vi "TEST_PP_Auto_Read.vi"() -> ()   [LabVIEW 2023]
uses:
  <vilib>/Rock Robotics/WPI/ThirdParty/MJansen/PathPlanner/TypeDef/PathPlannerTrajectoryState.ctl
  <vilib>/Rock Robotics/WPI/ThirdParty/JAS_Junk/TrajLib/TypeDef/TRANSLATION2D.ctl
  <vilib>/Rock Robotics/WPI/ThirdParty/JAS_Junk/TrajLib/TypeDef/ROTATION2D.ctl
  <vilib>/Rock Robotics/WPI/ThirdParty/MJansen/PathPlanner/TypeDef/PathPlannerPathConstraints.ctl
  <vilib>/Rock Robotics/WPI/ThirdParty/MJansen/PathPlanner/TypeDef/PathPlannerCommandUtil.ctl
  <vilib>/Rock Robotics/WPI/ThirdParty/MJansen/PathPlanner/ENum/PathPlanner_CommandUtilType_ENUM.ctl
  <vilib>/Rock Robotics/WPI/ThirdParty/MJansen/PathPlanner/TypeDef/PathPlannerEventMarker.ctl
  <vilib>/Rock Robotics/WPI/ThirdParty/JAS_Junk/TrajLib/VI/Util_GetTime_U32.vi
  <vilib>/Rock Robotics/WPI/ThirdParty/JAS_Junk/TrajLib/VI/BoolCmd_Recv_Internal.vi
  <vilib>/Utility/error.llb/Clear Errors.vi
  <vilib>/Rock Robotics/WPI/ThirdParty/JAS_Junk/TrajLib/Pose2d_New_TRRO.vi
  <vilib>/Rock Robotics/WPI/ThirdParty/MJansen/PathPlanner/VI/PathPlanner_EventMarker_ShouldTrigger.vi
  <vilib>/Rock Robotics/WPI/ThirdParty/JAS_Junk/TrajLib/VI/BoolCmd_ObtainQueue.vi
  <vilib>/Rock Robotics/WPI/ThirdParty/JAS_Junk/TrajLib/Translation2d_GetDistance.vi
  <vilib>/Rock Robotics/WPI/ThirdParty/JAS_Junk/TrajLib/Pose2d_getTranslation.vi
  <vilib>/Rock Robotics/WPI/ThirdParty/JAS_Junk/TrajLib/Util_CalcDist.vi
  <vilib>/Rock Robotics/WPI/ThirdParty/JAS_Junk/TrajLib/VI/Util_GetTime_U64.vi
  <vilib>/Rock Robotics/Network Tables/NT Write Number.vi
  <vilib>/Rock Robotics/Network Tables/NT Read Number.vi
  <vilib>/Rock Robotics/WPI/ThirdParty/MJansen/PathPlanner/PathPlanner24.lvlib
  <vilib>/Rock Robotics/WPI/ThirdParty/JAS_Junk/TrajLib/Trajectory_Library.lvlib
panel:
  out "time":dbl
  out "FPGA_Time_Seconds":dbl
  out "pathName":string
  out "size(s)":i32
  out "#Shoot":dbl
  out "EventMarkers":T1[](array[typedef]) {"lastRobotPos"."Y" format="%14.3f"; "lastRobotPos"."X" format="%14.3f"; "markerPos"."Y" format="%14.3f"; "markerPos"."X" format="%14.3f"}
  out "Req_Shoot_2":bool
  out "Req_Shoot_1":bool
  out "Auto Command":T3
  out "PathPlannerState":T5={"TimeSeconds"=0.0, "VelocityMPS"=0.0, "AccerationMpsSq"=0.0, "HeadingAngularVelRadPerSec"=0.0, "PositionMeters"={"X"=0.0, "Y"=1.0}, "Heading"={"VALUE"=0.0, "COS"=1.0, "SIN"=0.0}, "TargetHolonomicRotation"={"VALUE"=0.0, "COS"=1.0, "SIN"=0.0}, "CurvatureRadPerMeter"=0.0, "PathPlannerConstraints"={"MaxVelocityMps;"=0.0, "MaxAccelerationMpsSq;"=0.0, "MaxAngularVelRadPsEc;"=0.0, "MaxAngularAccRadPSecSq"=0.0, "Exists"=FALSE}, "DeltaPos"=0.0} {"TargetHolonomicRotation"."SIN" format="%13.4f"; "TargetHolonomicRotation"."COS" format="%13.4f"; "TargetHolonomicRotation"."VALUE" format="%13.4f"; "Heading"."SIN" format="%13.4f"; "Heading"."COS" format="%13.4f"; "Heading"."VALUE" format="%13.4f"; "PositionMeters"."Y" format="%14.3f"; "PositionMeters"."X" format="%14.3f"}
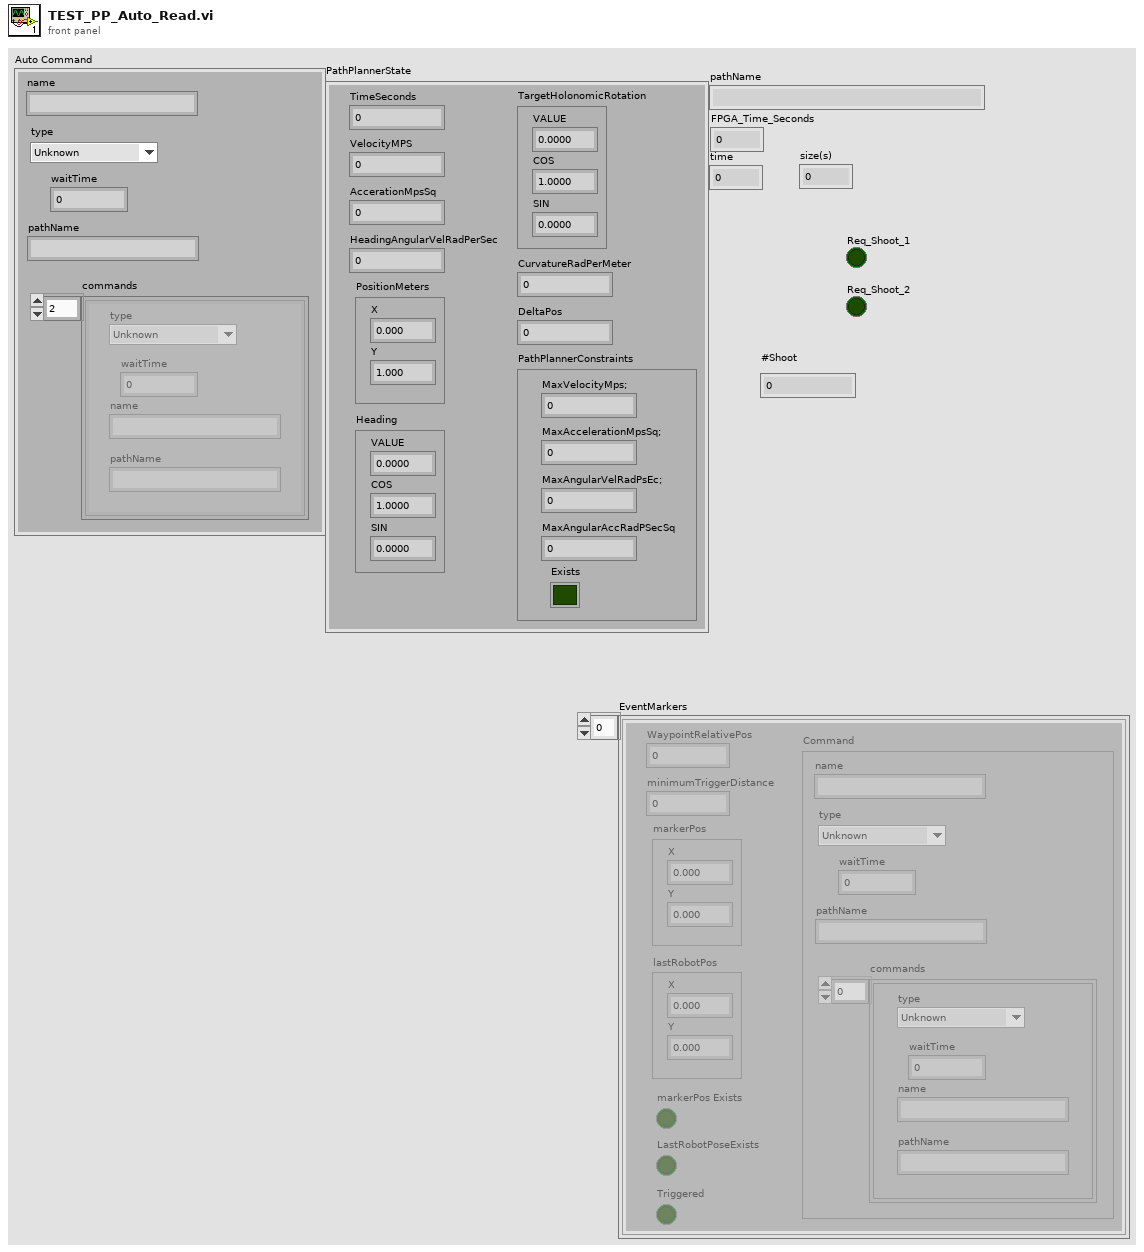
[diagram p1: front panel]
types:
  T1 = typedef "PathPlanner24.lvlib/PathPlannerEventMarker.ctl" = cluster{"WaypointRelativePos":dbl, "minimumTriggerDistance":dbl, "markerPos":T2, "lastRobotPos":T2, "Command":T3, "markerPos Exists":bool, "LastRobotPoseExists":bool, "Triggered":bool}
  T2 = typedef "Trajectory_Library.lvlib/TRANSLATION2D.ctl" = cluster{"X":dbl, "Y":dbl}
  T3 = typedef "PathPlanner24.lvlib/PathPlannerCommandUtil.ctl" = cluster{"waitTime":dbl, "name":string, "pathName":string, "commands":cluster{"type":T4, "waitTime":dbl, "name":string, "pathName":string}[], "type":T4}
  T4 = typedef "PathPlanner24.lvlib/PathPlanner_CommandUtilType_ENUM.ctl" = enum16{"Unknown", "Wait", "Named", "Path", "Sequential", "Parallel", "Race", "Deadline"}
  T5 = typedef "PathPlanner24.lvlib/PathPlannerTrajectoryState.ctl" = cluster{"TimeSeconds":dbl, "VelocityMPS":dbl, "AccerationMpsSq":dbl, "HeadingAngularVelRadPerSec":dbl, "PositionMeters":T2, "Heading":T6, "TargetHolonomicRotation":T6, "CurvatureRadPerMeter":dbl, "PathPlannerConstraints":T7, "DeltaPos":dbl}
  T6 = typedef "Trajectory_Library.lvlib/ROTATION2D.ctl" = cluster{"VALUE":dbl, "COS":dbl, "SIN":dbl}
  T7 = typedef "PathPlanner24.lvlib/PathPlannerPathConstraints.ctl" = cluster{"MaxVelocityMps;":dbl, "MaxAccelerationMpsSq;":dbl, "MaxAngularVelRadPsEc;":dbl, "MaxAngularAccRadPSecSq":dbl, "Exists":bool}
  T8 = cluster{"type":T4, "waitTime":dbl, "name":string, "pathName":string}[]
  T9 = typedef "PathPlanner24.lvlib/PathPlannerPath.ctl" = cluster{"BezierPoints":T2[], "PreviewStartingRotation":T6, "Reversed":bool, "RotationTargets":T10[], "ConstraintZones":T11[], "EventMarkers":T1[], "GlobalConstraints":T7, "GoalEndState":T12, "AllPoints":T13[]}
  T10 = typedef "PathPlanner24.lvlib/PathPlannerRotationTarget.ctl" = cluster{"target":T6, "WaypointRelativePosition":dbl, "Exists":bool}
  T11 = typedef "PathPlanner24.lvlib/PathPlannerConstraintsZone.ctl" = cluster{"minWaypointPos":dbl, "maxWaypointPos":dbl, "Constraints":T7, "Present":bool}
  T12 = typedef "PathPlanner24.lvlib/PathPlannerGoalEndState.ctl" = cluster{"Velocity":dbl, "Rotation":T6}
  T13 = typedef "PathPlanner24.lvlib/PathPlannerPathPoint.ctl" = cluster{"Position":T2, "HolonomicRotation":T6, "DistAlongPath":dbl, "CurveRadius":dbl, "MaxV":dbl, "Constraints":T7, "HolonomicRotationExists":bool}
  T14 = typedef "Trajectory_Library.lvlib/CHASSIS_SPEEDS.ctl" = cluster{"vX":dbl, "vY":dbl, "vOmega":dbl}
  T15 = typedef "PathPlanner24.lvlib/PathPlannerTrajectory.ctl" = cluster{"States":T5[]}
  T16 = typedef "Trajectory_Library.lvlib/POSE2D.ctl" = cluster{"TRANSLATION":T2, "ROTATION":T6}
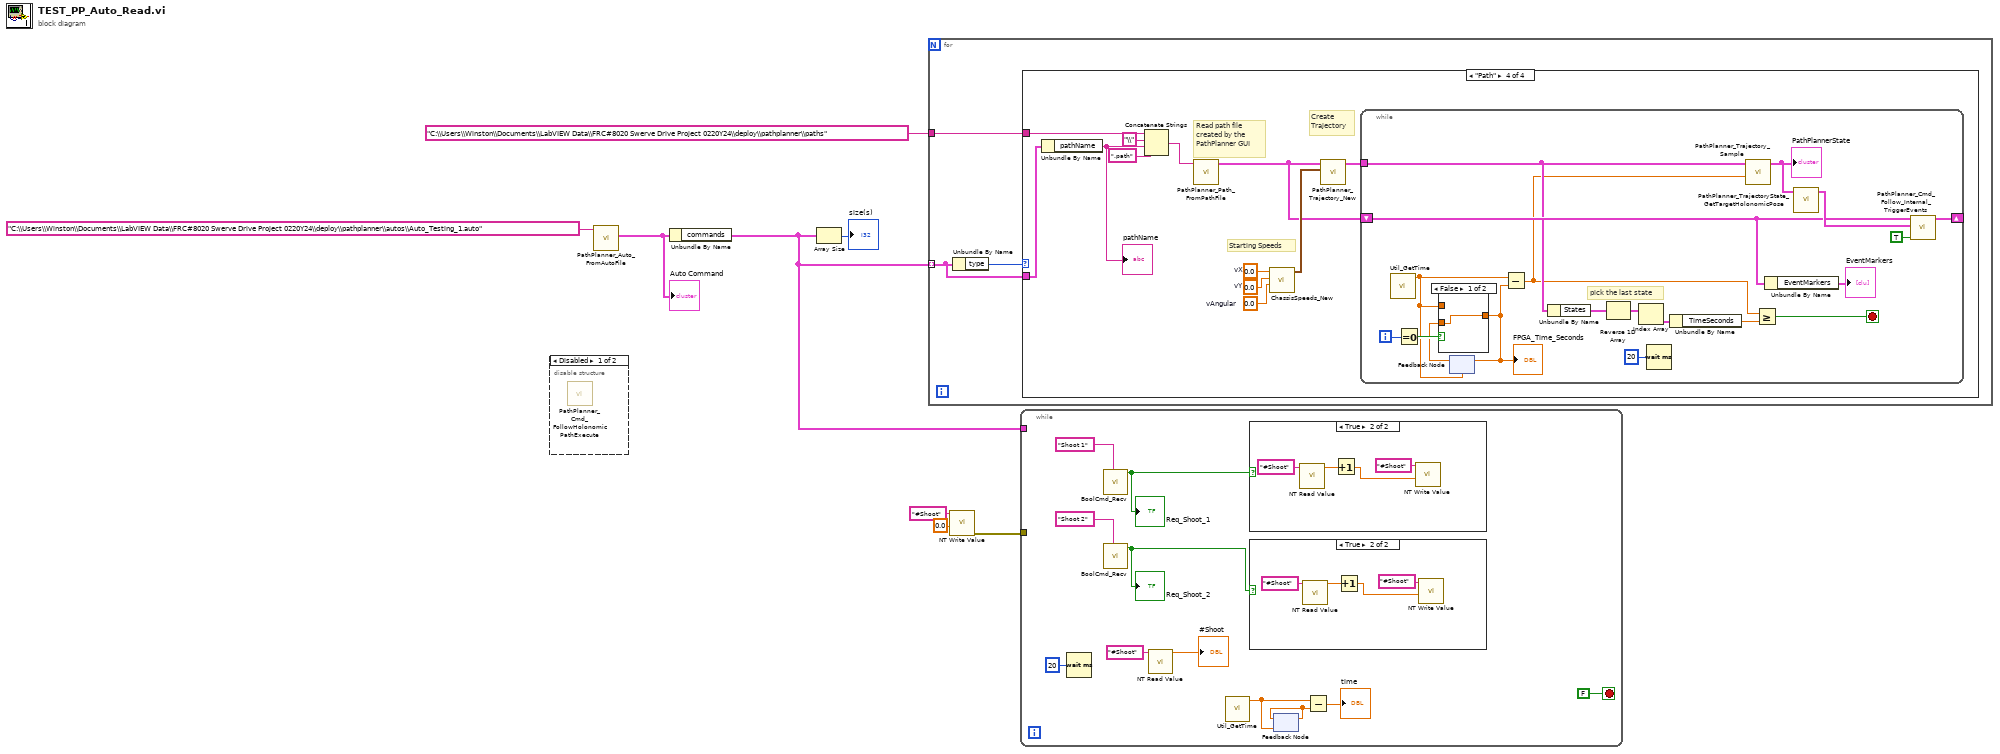
[diagram p0: block diagram]
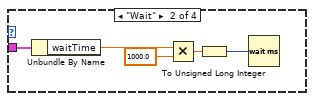
[diagram p3: hidden frame]
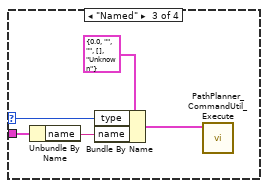
[diagram p4: hidden frame]
diagram:
  n1 = disable-structure shown="Disabled" {
    frame Disabled {
      n2 = call <vilib>:"PathPlanner_Cmd_FollowHolonomicPathExecute.vi"() -> ()  [unwired: 7 in, 5 out]
    }
    frame Enabled {
    }
  }
  n3 = call "PathPlanner_Auto_FromAutoFile.vi"("FileName"="C:\\Users\\Winston\\Documents\\LabVIEW Data\\FRC#8020 Swerve Drive Project 0220Y24\\deploy\\pathplanner\\autos\\Auto_Testing_1.auto") -> ("Auto Command"=w4:T3)  [unwired: 8 in, 2 out]
  "Auto Command" <- w4
  n4 = Unbundle By Name(w4) -> ("commands"=w1:T8)
  n5 = Array Size(array=w1) -> (size(s)=→"size(s)":i32)
  n6 = for {
    tunnel: w1 -> [w9] mode=indexing
    tunnel: "C:\\Users\\Winston\\Documents\\LabVIEW Data\\FRC#8020 Swerve Drive Project 0220Y24\\deploy\\pathplanner\\paths" ("FileName") -> [w10]
    n7 = Unbundle By Name(w9) -> ("type"=w11:T4)
    n8 = case shown="\"Path\"" w11 {
      selector: w11 -> [_ _ w19 _]
      tunnel: w10 -> [_ _ _ w27]
      tunnel: w9 -> [_ w16 w21 w26]
      frame "Unknown", Default {
      }
      frame "Wait" {
        n9 = Unbundle By Name(w16) -> ("waitTime"=w15:dbl)
        n10 = Multiply(x=w15, y=1000.0) -> (x*y=w13:dbl)
        n11 = To Unsigned Long Integer(number=w13) -> (unsigned 32bit integer=w12:u32)
        n12 = Wait (ms)(milliseconds to wait=w12) -> ()  [unwired: 1 out]
      }
      frame "Named" {
        n13 = Unbundle By Name(w21) -> ("name"=w18:string)
        n14 = Bundle By Name(cluster=T3 {"waitTime"=0.0, "name"="", "pathName"="", "commands"=[], "type"=enum."Unknown"} ("CommandUtil"), "type"=w19, "name"=w18) -> (w17:T3)
        n15 = call <vilib>:"PathPlanner_CommandUtil_Execute.vi"("Command"=w17) -> ()  [unwired: 11 in]
      }
      frame "Path" {
        w32 = 0.0  # vX
        w31 = 0.0  # vY
        w30 = 0.0  # vAngular
        # "Read path file\ncreated by the\nPathPlanner GUI"
        # "Create\nTrajectory"
        # "Starting Speeds"
        n16 = Unbundle By Name(w26) -> ("pathName"=w23:string)
        "pathName" <- w23
        n17 = Concatenate Strings(w27, "\\" ("string"), w23, ".path" ("string")) -> (w25:string)
        n18 = call <vilib>:"PathPlanner_Path_FromPathFile.vi"("FileName"=w25) -> ("PathPlannerPath"=w28:T9)  [unwired: 8 in, 2 out]
        n19 = call <vilib>:"ChassisSpeeds_New.vi"("vAngular"=w30, "vY"=w31, "vX"=w32) -> ("CHASSIS"=w33:T14)  [unwired: 8 in]
        n20 = call <vilib>:"PathPlanner_Trajectory_New.vi"("StartingSpeeds"=w33, "Path"=w28) -> ("PathPlannerTrajectory"=w29:T15)  [unwired: 9 in]
        n21 = while {
          tunnel: w29 -> [w45]
          shift-right: [w49] -> _
          shift-left: w28 -> [w47]
          i -> [w38]
          stop <- w39 stop-if-true
          # "pick the last state"
          n22 = call <vilib>:"Util_GetTime.vi"() -> ("FPGA_Time_Seconds"=w36:dbl)  [unwired: 9 in, 2 out]
          n23 = Equal To 0?(x=w38) -> (x = 0?=w37:bool)
          n24 = feedback #1(w36) -> (w34:dbl)
          n25 = case shown="False" w37 {
            tunnel: [w53 w54] -> w35
            tunnel: w36 -> [_ w54]
            tunnel: w34 -> [w53 _]
            frame False {
            }
            frame True {
            }
          }
          "FPGA_Time_Seconds" <- w35
          n26 = feedback-in #1(w35) -> ()
          n27 = Subtract(x=w36, y=w35) -> (x-y=w40:dbl)
          n28 = Unbundle By Name(w45) -> ("States"=w44:T5[])
          n29 = Reverse 1D Array(array=w44) -> (reversed array=w43:T5[])
          n30 = Index Array(array=w43) -> (element=w42:T5)  [unwired: 1 in]
          n31 = Wait (ms)(milliseconds to wait=u32 20) -> ()  [unwired: 1 out]
          n32 = Unbundle By Name(w42) -> ("TimeSeconds"=w41:dbl)
          n33 = call <vilib>:"PathPlanner_Trajectory_Sample.vi"("Time"=w40, "PathPlannerTrajectory"=w45) -> ("PathPlannerState"=w46:T5)  [unwired: 9 in]
          "PathPlannerState" <- w46
          n34 = Greater Or Equal?(x=w40, y=w41) -> (x >= y?=w39:bool)
          n35 = Unbundle By Name(w47) -> ("EventMarkers"=→"EventMarkers":T1[])
          n36 = call <vilib>:"PathPlanner_TrajectoryState_GetTargetHolonomicPose.vi"("PathPlannerState"=w46) -> ("TargetHolonomicPose"=w50:T16)  [unwired: 10 in]
          n37 = call <vilib>:"PathPlanner_Cmd_Follow_Internal_TriggerEvents.vi"("TrigerEvents"=TRUE, "Current Pose SI"=w50, "RePlannedPath in"=w47) -> ("RePlannedPath out"=w49:T9)  [unwired: 8 in]
        }
      }
    }
  }
  n38 = call-poly <vilib>:"NT Write Value.vi"("value"=0.0, "name"="#Shoot") -> ("error out"=w5:errorcluster)  [unwired: 9 in]
  n39 = while {
    tunnel: w5 -> [_]
    tunnel: w1 -> [_]
    stop <- FALSE stop-if-true
    n40 = Wait (ms)(milliseconds to wait=u32 20) -> ()  [unwired: 1 out]
    n41 = call <vilib>:"BoolCmd_Recv.vi"("Command Name"="Shoot 1") -> ("New Request"=w61:bool)  [unwired: 9 in, 1 out]
    "Req_Shoot_1" <- w61
    n42 = call <vilib>:"BoolCmd_Recv.vi"("Command Name"="Shoot 2") -> ("New Request"=w60:bool)  [unwired: 9 in, 1 out]
    "Req_Shoot_2" <- w60
    n43 = call-poly <vilib>:"NT Read Value.vi"("name"="#Shoot") -> ("value"=→"#Shoot":dbl)  [unwired: 8 in, 2 out]
    n44 = call <vilib>:"Util_GetTime.vi"() -> ("FPGA_Time_Seconds"=w56:dbl)  [unwired: 9 in, 2 out]
    n45 = case shown="True" w61 {
      frame False {
      }
      frame True {
        n46 = call-poly <vilib>:"NT Read Value.vi"("name"="#Shoot") -> ("value"=w71:dbl)  [unwired: 8 in, 2 out]
        n47 = Increment(x=w71) -> (x+1=w70:dbl)
        n48 = call-poly <vilib>:"NT Write Value.vi"("value"=w70, "name"="#Shoot") -> ()  [unwired: 9 in, 1 out]
      }
    }
    n49 = case shown="True" w60 {
      frame False {
      }
      frame True {
        n50 = call-poly <vilib>:"NT Read Value.vi"("name"="#Shoot") -> ("value"=w67:dbl)  [unwired: 8 in, 2 out]
        n51 = Increment(x=w67) -> (x+1=w66:dbl)
        n52 = call-poly <vilib>:"NT Write Value.vi"("value"=w66, "name"="#Shoot") -> ()  [unwired: 9 in, 1 out]
      }
    }
    n53 = feedback #2(w56) -> (w57:dbl)
    n54 = feedback-in #2(w57) -> ()
    n55 = Subtract(x=w56, y=w57) -> (x-y=→"time":dbl)
  }
